vi "Test_Boolean.vi"(8 "error in (no error)":errorcluster, 10 "Parameters":string, 11 "reference in":refnum<class "Test_Sim.lvclass">) -> (0 "error out":errorcluster, 2 "Result":bool, 3 "reference in":refnum<class "Test_Sim.lvclass">)   [LabVIEW 2020, in "Test_Sim.lvlib" / "Test_Sim.lvclass"]
uses:
  Test_Sim.lvclass
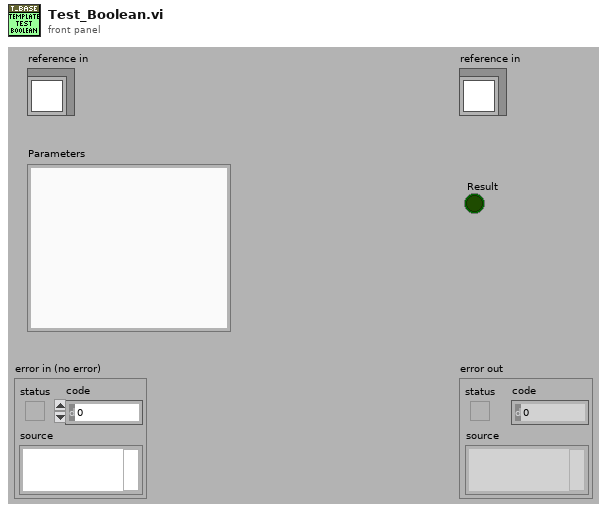
[diagram p1: front panel]
types:
  T1 = typedef "Test_Sim.lvlib/Test_Sim.lvclass/ObjectAttributes.ctl" = cluster{"Config":T2}
  T2 = typedef "Test_Sim.lvlib/Test_Sim.lvclass/Config.ctl" = cluster{"_default":string}
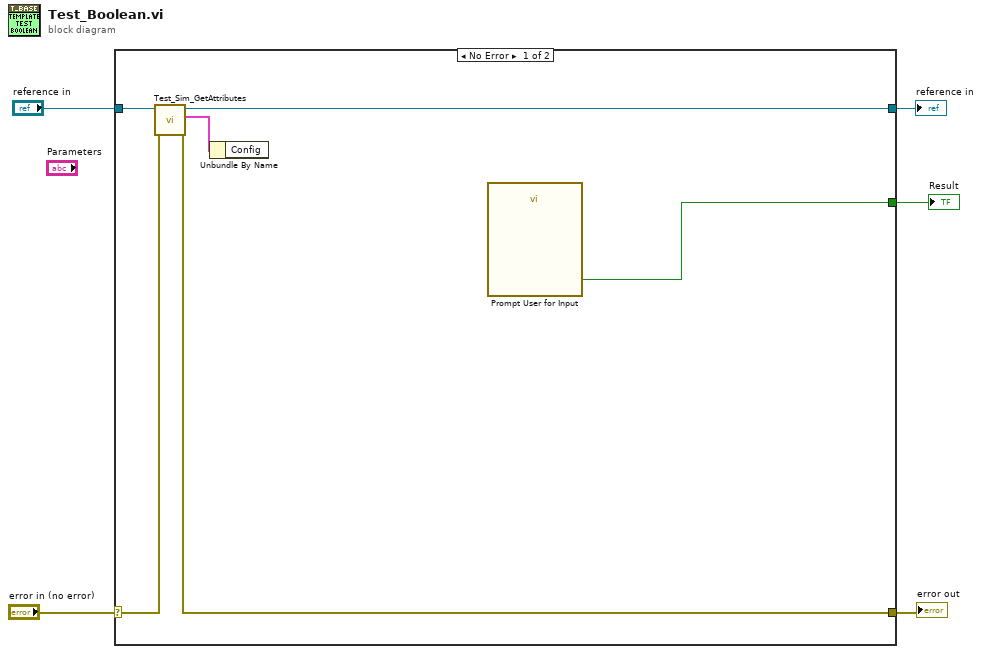
[diagram p0: block diagram]
diagram:
  n1 = case shown="No Error" "error in (no error)" {
    selector: "error in (no error)" -> [w11 w13]
    tunnel: [w9 w13] -> w4
    tunnel: [w7 w12] -> w2
    tunnel: "reference in" -> [w8 w12]
    tunnel: [w6 _] -> w1
    frame No Error {
      n2 = call "Test_Sim_GetAttributes.vi"("error in (no error)"=w11, "reference in"=w8) -> ("error out"=w9:errorcluster, "Data"=w10:T1, "reference out"=w7:refnum<class "Test_Sim.lvclass">)  [unwired: 6 in, 1 out]
      n3 = Unbundle By Name(w10) -> ()  [unwired: 1 out]
      n4 = call "Prompt User for Input"() -> ("Value"=w6:bool)  [unwired: 17 in, 2 out]
    }
    frame Error {
    }
  }
  "error out" <- w4
  "reference in" <- w2
  "Result" <- w1
